vi "RichToFlatnixnet_grpc_WriteSignalWaveformRequest.vi"(5 "OutputClusterType":T1, 11 "InputCluster":T4) -> (3 "OutputCluster":T1)   [LabVIEW 2025, in "xnet-grpc_client.lvlib"]
uses:
  xnet-grpc_client.lvlib
  nixnet_grpc_WriteSignalWaveformRequest.ctl
  nixnet_grpc_WriteSignalWaveformRequest_timeout_enum/nixnet_grpc_WriteSignalWaveformRequest_timeout_enum.lvclass
  nidevice_grpc_Session.ctl
  nixnet_grpc_WriteSignalWaveformRequest_Flat.ctl
  nidevice_grpc_Session_Flat.ctl
  nixnet_grpc_TimeOut.ctl
  nixnet_grpc_WriteSignalWaveformRequest_timeout_enum/nixnet_grpc_WriteSignalWaveformRequest_timeout_enum.lvclass/nixnet_grpc_WriteSignalWaveformRequest_timeout_enum.ctl
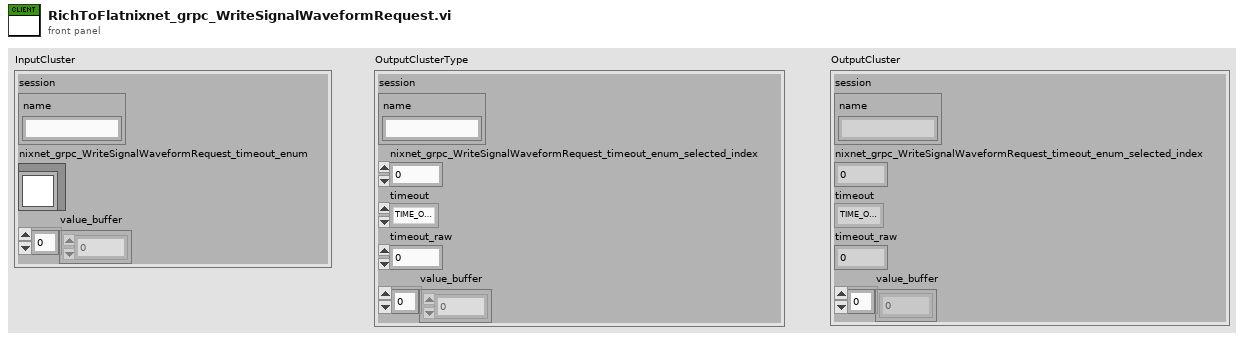
[diagram p1: front panel]
types:
  T1 = typedef "xnet-grpc_client.lvlib/nixnet_grpc_WriteSignalWaveformRequest_Flat.ctl" = cluster{"session":T2, "nixnet_grpc_WriteSignalWaveformRequest_timeout_enum_selected_index":i32, "timeout":T3, "timeout_raw":dbl, "value_buffer":dbl[]}
  T2 = typedef "xnet-grpc_client.lvlib/nidevice_grpc_Session_Flat.ctl" = cluster{"name":string}
  T3 = typedef "xnet-grpc_client.lvlib/nixnet_grpc_TimeOut.ctl" = enum32{"TIME_OUT_NONE", "TIME_OUT_INFINITE"}
  T4 = typedef "xnet-grpc_client.lvlib/nixnet_grpc_WriteSignalWaveformRequest.ctl" = cluster{"session":T5, "nixnet_grpc_WriteSignalWaveformRequest_timeout_enum":refnum<class "nixnet_grpc_WriteSignalWaveformRequest_timeout_enum.lvclass">, "value_buffer":dbl[]}
  T5 = typedef "xnet-grpc_client.lvlib/nidevice_grpc_Session.ctl" = cluster{"name":string}
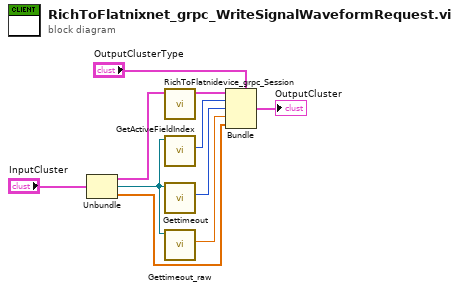
[diagram p0: block diagram]
diagram:
  n1 = Unbundle "Unbundle"("InputCluster") -> ("session"=w7:T5, "nixnet_grpc_WriteSignalWaveformRequest_timeout_enum"=w5:refnum<class "nixnet_grpc_WriteSignalWaveformRequest_timeout_enum.lvclass">, "value_buffer"=w1:dbl[])
  n2 = call "RichToFlatnidevice_grpc_Session.vi"("InputCluster"=w7) -> ("OutputCluster"=w6:T2)  [unwired: 10 in]
  n3 = call "GetActiveFieldIndex.vi"("OneOfTemplate in"=w5) -> ("Active Field Index"=w4:i32)  [unwired: 8 in, 2 out]
  n4 = call "Gettimeout.vi"("OneOfTemplate in"=w5) -> ("Get_Val"=w3:T3)  [unwired: 8 in, 2 out]
  n5 = call "Gettimeout_raw.vi"("OneOfTemplate in"=w5) -> ("Get_Val"=w2:dbl)  [unwired: 8 in, 2 out]
  n6 = Bundle "Bundle"(cluster="OutputClusterType", "session"=w6, "nixnet_grpc_WriteSignalWaveformRequest_timeout_enum_selected_index"=w4, "timeout"=w3, "timeout_raw"=w2, "value_buffer"=w1) -> (→"OutputCluster":T1)
